vi "External Data.vi"(8 "error in (no error)":errorcluster, 10 "Pipeline In":refnum<queue>, 11 "External Queue In":refnum<queue>) -> (0 "error out":errorcluster)   [LabVIEW 2016]
uses:
  Message Format.ctl
  StateDef_generic.ctl
  <vilib>/DAQmx/read.llb/DAQmx Read (Analog 1D Wfm NChan NSamp).vi
  <vilib>/DAQmx/miscellaneous.llb/DAQmx Fill In Error Info.vi
panel:
  out "External Sensors":T1
  in  "samples per read":i32=100
  # "EXTERNAL SENSORS"
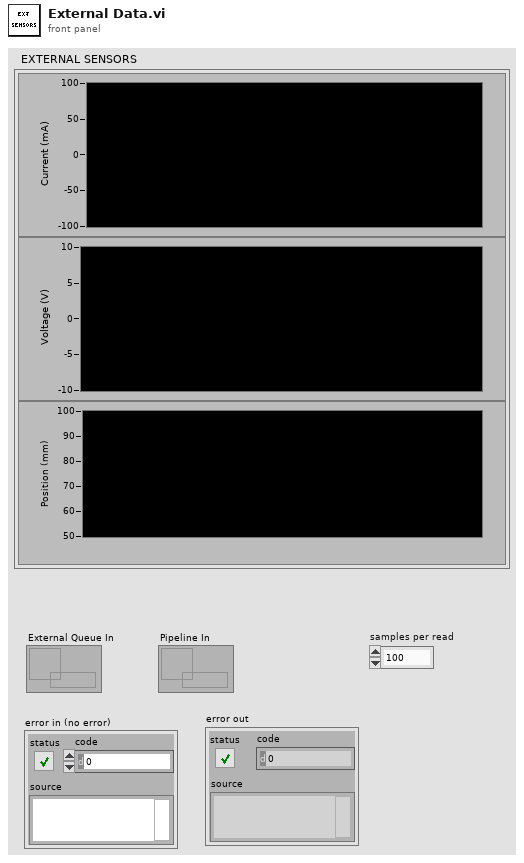
[diagram p1: front panel]
types:
  T1 = cluster{"Waveform Chart":waveform(dbl), "Waveform Chart 2":waveform(dbl), "Waveform Chart 3":waveform(dbl)}
  T2 = typedef "StateDef_generic.ctl" = enum16{"Initialize", "Running", "Exit"}
  T3 = typedef "Message Format.ctl" = cluster{"header":string, "data":variant}
  T4 = cluster{"Waveform":waveform(dbl), "Waveform":waveform(dbl), "Waveform":waveform(dbl)}
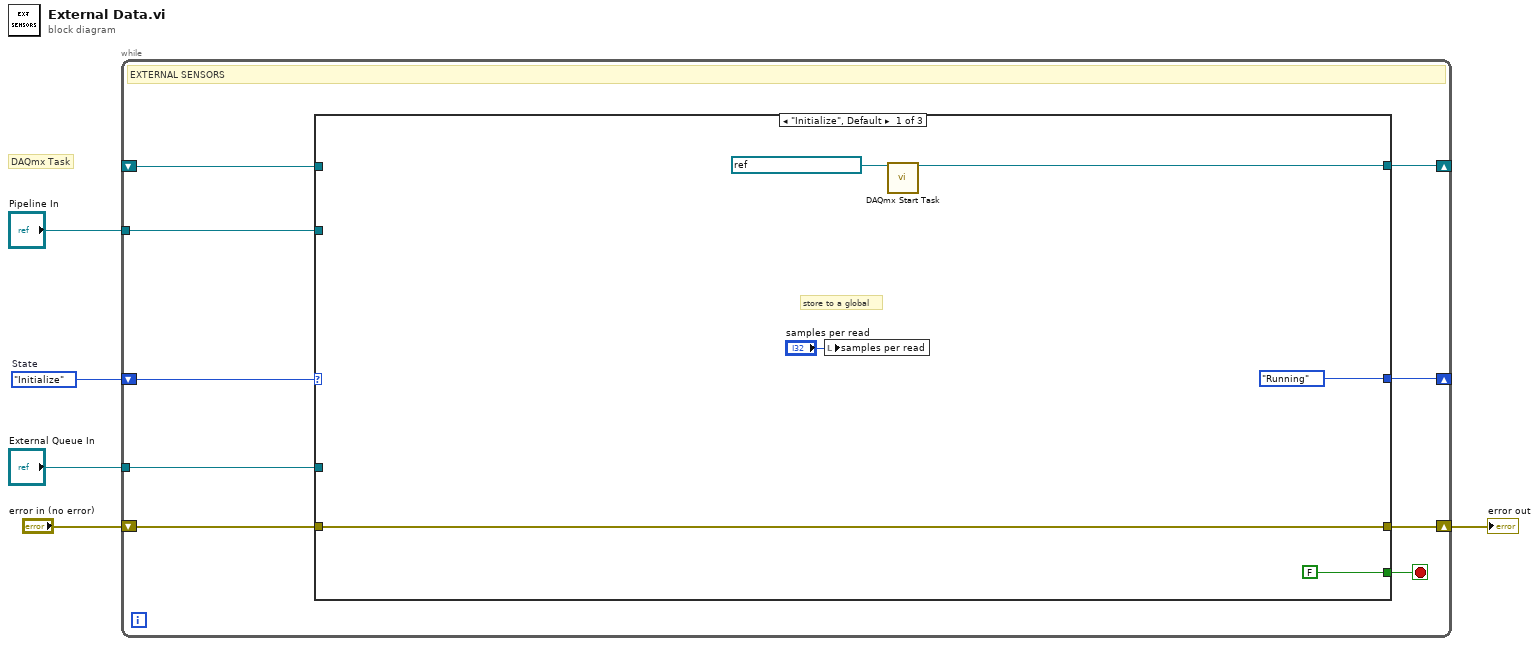
[diagram p0: block diagram]
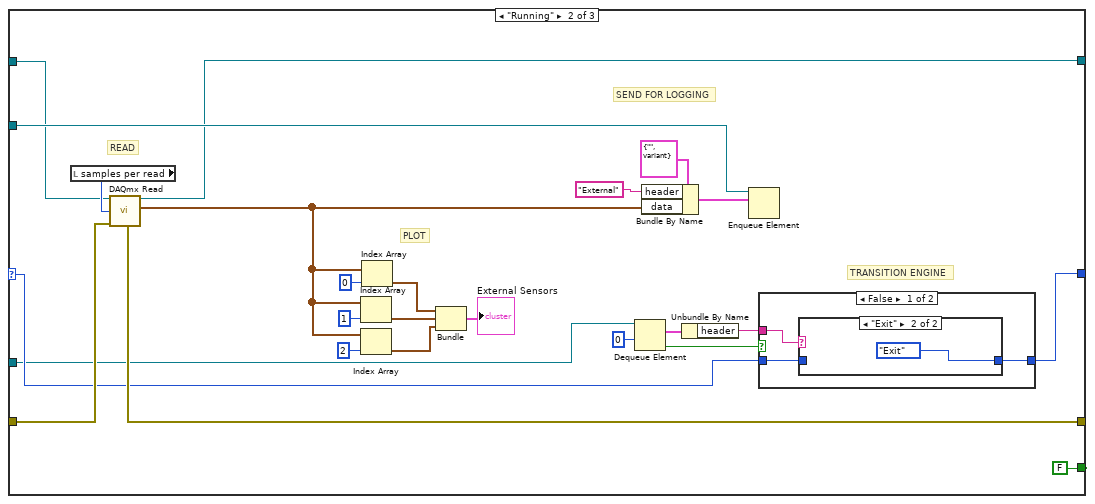
[diagram p2: hidden frame]
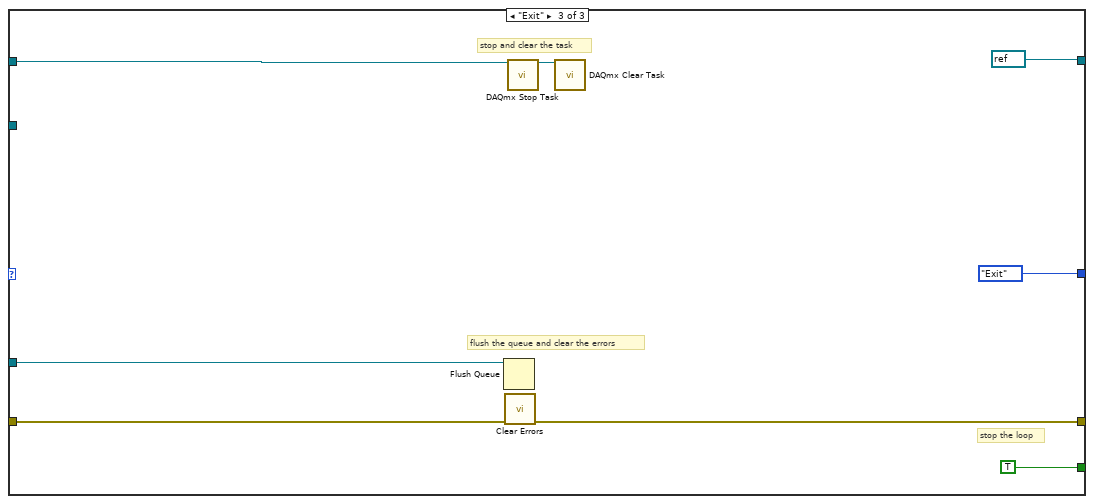
[diagram p5: hidden frame]
diagram:
  w3 = StateDef_generic."Initialize"  # State
  # "DAQmx Task"
  n1 = while {
    shift-right: [w6] -> w1
    shift-left: "error in (no error)" -> [w7]
    shift-right: [w9] -> _
    shift-left: _ -> [w13]
    tunnel: "Pipeline In" -> [w12]
    shift-right: [w8] -> _
    shift-left: w3 -> [w11]
    tunnel: "External Queue In" -> [w10]
    stop <- w14 stop-if-true
    # "EXTERNAL SENSORS"
    n2 = case shown="\"Initialize\", Default" w11 {
      selector: w11 -> [_ w25 _]
      tunnel: [FALSE FALSE TRUE] -> w14
      tunnel: w13 -> [_ w22 w55]
      tunnel: w12 -> [_ w42 _]
      tunnel: w10 -> [_ w21 w54]
      tunnel: [w18 w23 refnum<k21> refnum ("task out")] -> w9
      tunnel: [StateDef_generic."Running" ("State") w24 StateDef_generic."Exit" ("State")] -> w8
      tunnel: w7 -> [w16 w32 w53]
      tunnel: [w16 w31 w52] -> w6
      frame "Initialize", Default {
        # "store to a global"
        n3 = local write "samples per read"("samples per read") -> ()
        n4 = call <vilib>:"DAQmx Start Task.vi"("task/channels in"=refnum<k21> "mass-shifter external" ("DAQmx Task Name")) -> ("task out"=w18:refnum<k21>)  [unwired: 13 in, 1 out]
      }
      frame "Running" {
        # "TRANSITION ENGINE"
        # "PLOT"
        # "SEND FOR LOGGING"
        # "READ"
        n5 = local read "samples per read"() -> (w45:i32)
        n6 = call-poly <vilib>:"DAQmx Read.vi"("task/channels in"=w22, "number of samples per channel"=w45, "error in"=w32) -> ("task out"=w23:refnum<k21>, "data"=w37:waveform(dbl)[], "error out"=w31:errorcluster)  [unwired: 10 in]
        n7 = Index Array(array=w37, index=1) -> (element=w35:waveform(dbl))
        n8 = Index Array(array=w37, index=2) -> (element=w34:waveform(dbl))
        n9 = Index Array(array=w37, index=0) -> (element=w36:waveform(dbl))
        n10 = Bundle("Waveform"=w36, "Waveform"=w35, "Waveform"=w34) -> (→"External Sensors":T4)  [unwired: 1 in]
        n11 = Dequeue Element(queue=w21, timeout in ms (-1)=0) -> (element=w27:T3, timed out?=w28:bool)  [unwired: 1 in, 2 out]
        n12 = Bundle By Name(cluster=T3 {"header"="", "data"=variant} ("msg format"), "header"="External", "data"=w37) -> (w41:T3)
        n13 = Unbundle By Name(w27) -> ("header"=w26:string)
        n14 = Enqueue Element(queue=w42, element=w41) -> ()  [unwired: 2 in, 3 out]
        n15 = case shown="False" w28 {
          tunnel: w25 -> [w46 w51]
          tunnel: w26 -> [w48 _]
          tunnel: [w47 w51] -> w24
          frame False {
            n16 = case shown="\"Exit\"" w48 {
              tunnel: [w49 StateDef_generic."Exit" ("State")] -> w47
              tunnel: w46 -> [w49 _]
              frame "any other", Default {
              }
              frame "Exit" {
              }
            }
          }
          frame True {
          }
        }
      }
      frame "Exit" {
        # "stop and clear the task"
        # "stop the loop"
        # "flush the queue and clear the errors"
        n17 = Flush Queue(queue=w54) -> ()  [unwired: 1 in, 3 out]
        n18 = call <vilib>:"Clear Errors.vi"("error in (no error)"=w53) -> ("error out"=w52:errorcluster)  [unwired: 5 in, 1 out]
        n19 = call <vilib>:"DAQmx Stop Task.vi"("task/channels in"=w55) -> ("task out"=w58:refnum<k21>)  [unwired: 13 in, 1 out]
        n20 = call <vilib>:"DAQmx Clear Task.vi"("task in"=w58) -> ()  [unwired: 14 in, 1 out]
      }
    }
  }
  "error out" <- w1
